vi "getDataLine.vi"(8 "error in":T1, 9 "FullOnly":bool=TRUE, 10 "length":i32, 11 "channel":i32) -> (0 "error out":T1, 2 "Unit value":string, 3 "linearray":sgl[](array[numeric]))   [LabVIEW 2016]
doc: "Like the getData.vi this VI processes data. But it has been created only for the lineView. The in- and outputs are quite similar to getData.vi.\nThe number of data points in the linearray can be modified by the user by changing the input \"length\"."
uses:
  Controls/Error_Out.ctl
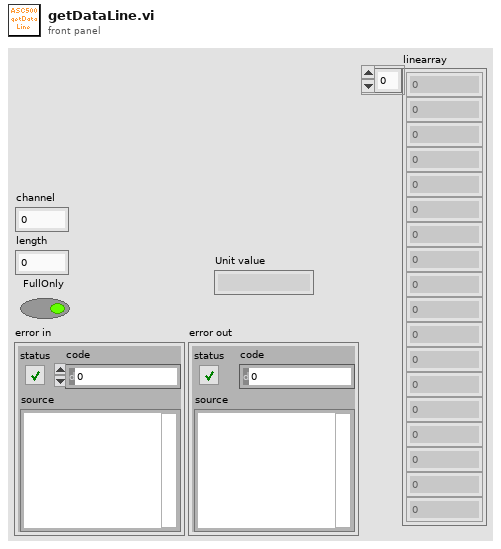
[diagram p1: front panel]
types:
  T1 = typedef "Error_Out.ctl" = errorcluster
  T2 = typedef "Metadata-Cluster.ctl" = cluster{"DYB_Order":i32, "Spalte":i32, "Zeile":i32, "Abstand Datenpunkte":dbl, "Abstand Scanzeilen":dbl, "x-Koordinate 1. Punkt":dbl, "y-Koordinate 2. Punkt":dbl, "Neigungswinkel Scanfeld":dbl, "Einheit Variablen":i32, "stepVal":dbl, "stepValNum":dbl, "offsetVal":dbl, "unitVal":i32}
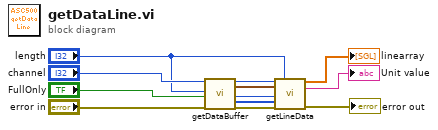
[diagram p0: block diagram]
diagram:
  n1 = call "getDataBuffer.vi"("channel"="channel", "dataSize_in"="length", "FullOnly"="FullOnly", "error in"="error in") -> ("dataSize"=w2:i32, "meta"=w3:T2, "frameNo"=w4:i32, "data"=w5:i32[], "error out"=w6:T1)  [unwired: 10 in, 1 out]
  n2 = call "getLineData.vi"("index"=w2, "length"="length", "meta"=w3, "frameNO"=w4, "data"=w5, "error in"=w6) -> ("linearray"=→"linearray":sgl[], "Unit value"=→"Unit value":string, "error out"=→"error out":T1)  [unwired: 7 in]
